vi "ImageSelectLine.vi"(11 "Image":T2) -> (3 "selectedLine":i16[](array[numeric]))   [LabVIEW 2021]
uses:
  <vilib>/vision/Image Controls.llb/IMAQ Image.ctl
  <vilib>/userdefined/High Color/IMAQdx.ctl
panel:
  in  "Session in":T1
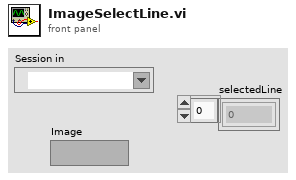
[diagram p1: front panel]
types:
  T1 = typedef "IMAQdx.ctl" = refnum<k21>
  T2 = typedef "IMAQ Image.ctl" = refnum<image>
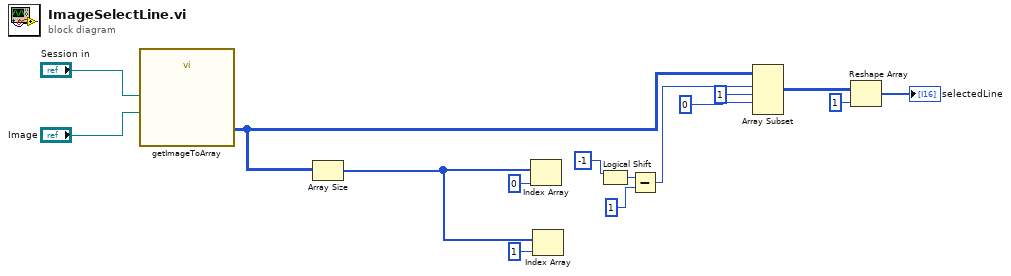
[diagram p0: block diagram]
diagram:
  n1 = call "getImageToArray.vi"("New Image"="Image", "Session in"="Session in") -> ("imageGrayArray"=w3:u16[][])  [unwired: 9 in]
  n2 = Array Size(array=w3) -> (size(s)=w1:i32[])
  n3 = Index Array(array=w1, index=0) -> ()  [unwired: 1 out]
  n4 = Index Array(array=w1, index=1) -> ()  [unwired: 1 out]
  n5 = Logical Shift(y=-1 ("x")) -> (x << y=w12:i32)  [unwired: 1 in]
  n6 = Subtract(x=w12, y=1) -> (x-y=w13:i32)
  n7 = Array Subset(array=w3, index (row)=w13, length (row)=1 ("length"), index (col)=0 ("index")) -> (w7:u16[][])  [unwired: 1 in]
  n8 = Reshape Array(w7, 1 ("dimension size")) -> (→"selectedLine":u16[])
